vi "Get Ordered Channels_Status_IO.vi"(8 "error in (no error)":errorcluster, 11 "IO in":refnum<class "IO.lvclass">) -> (0 "error out":errorcluster, 1 "Ordered ICP2-DI Channels":T3[](array[typedef]), 2 "Ordered ICP2-DO Channels":T2[](array[typedef]), 3 "IO out":refnum<class "IO.lvclass">, 4 "Ordered ICP1-DO Channels":T1[](array[typedef]))   [LabVIEW 2022 SP3]
uses:
  IO.lvclass
  Typedefs/ICP2-DO Channel Names.ctl
  Typedefs/ICP2-DI Channel Names.ctl
  Typedefs/ICP1-D0 Channel Names.ctl
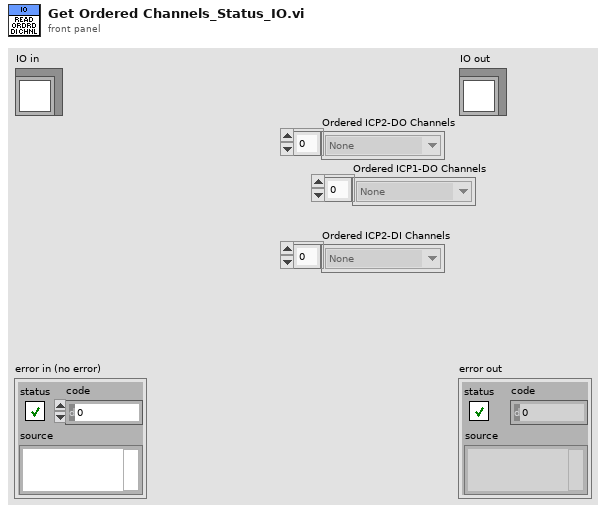
[diagram p1: front panel]
types:
  T1 = typedef "IO.lvclass/ICP1-D0 Channel Names.ctl" = enum16{"None", "Meniscus Pressure Reg PWR - R1", "Meniscus Pressure Reg PWR - R2", "Meniscus Pressure Reg PWR - R3", "Meniscus Pressure Reg PWR - R4", "Meniscus Pressure Reg PWR - R5", "Meniscus Pressure Reg PWR - R6", "Purge Valve Open - R1", "Purge Valve Open - R2", "Purge Valve Open - R3", "Purge Valve Open - R4", "Purge Valve Open - R5", "Purge Valve Open - R6"}
  T2 = typedef "IO.lvclass/ICP2-DO Channel Names.ctl" = enum16{"None", "Meniscus Valve Open - R1", "Meniscus Valve Open - R2", "Meniscus Valve Open - R3", "Meniscus Valve Open - R4", "Meniscus Valve Open - R5", "Meniscus Valve Open - R6", "Ink Flow Valve Open - R1", "Ink Flow Valve Open - R2", "Ink Flow Valve Open - R3", "Ink Flow Valve Open - R4", "Ink Flow Valve Open - R5", "Ink Flow Valve Open - R6", "SW_LED - Ink Valve - R1", "SW_LED - Ink Valve - R2", "SW_LED - Ink Valve - R3", "Recirc Pump On - R1", "Recirc Pump On - R2", "Recirc Pump On - R3", "Recirc Pump On - R4", "Recirc Pump On - R5", "Recirc Pump On - R6", "SW_LED - Ink Valve - R4", "SW_LED - Ink Valve - R5", "SW_LED - Ink Valve - R6"}
  T3 = typedef "IO.lvclass/ICP2-DI Channel Names.ctl" = enum16{"None", "SW - Ink Valve - R1", "SW - Ink Valve - R2", "SW - Ink Valve - R3", "SW - Ink Valve - R4", "SW - Ink Valve - R5", "SW - Ink Valve - R6", "SW - COVER INPUT SIDE", "SW - COVER OUTPUT SIDE", "SW - Purge - R1", "SW - Purge - R2", "SW - Purge - R3", "SW - Purge - R4", "SW - Purge - R5", "SW - Purge - R6"}
  T4 = typedef "IO.lvclass/Private Data.ctl" = cluster{"UserEvents":T5, "All Dependencies":cluster{"Class References":refnum<class>[], "Class Names":string[]}, "Status":T6}
  T5 = typedef "IO.lvclass/UserEvents.ctl" = cluster{"API Incoming Event":refnum<user-event>, "API Executed Event":refnum<user-event>, "API Return Event":refnum<user-event>, "Status Changed Event":refnum<user-event>}
  T6 = typedef "IO.lvclass/Status Cluster.ctl" = cluster{"Device Data":variant, "Ordered ICP1-DO Channels":T1[], "Ordered ICP2-DI Channels":T3[], "Ordered ICP2-DO Channels":T2[], "Ordered ICP1-AI Channels":T7[], "Ordered ICP1-AO Channels":T8[], "Ordered ICP2-AO Channels":T9[]}
  T7 = typedef "IO.lvclass/ICP1-AI Channel Names.ctl" = enum16{"None", "Meniscus Pressure Read - R1", "Meniscus Pressure Read - R2", "Meniscus Pressure Read - R3", "Meniscus Pressure Read - R4", "Meniscus Pressure Read - R5", "Meniscus Pressure Read - R6", "Meniscus Pressure Set - R1", "Meniscus Pressure Set - R2", "Meniscus Pressure Set - R3", "Meniscus Pressure Set - R4", "Meniscus Pressure Set - R5", "Meniscus Pressure Set - R6"}
  T8 = typedef "IO.lvclass/ICP1-AO Channel Names.ctl" = enum16{"None", "Meniscus Pressure Set - R1", "Meniscus Pressure Set - R2", "Meniscus Pressure Set - R3", "Meniscus Pressure Set - R4", "Meniscus Pressure Set - R5", "Meniscus Pressure Set - R6"}
  T9 = typedef "IO.lvclass/ICP2-AO Channel Names.ctl" = enum16{"None", "Recirc Pump Flow Set - R1", "Recirc Pump Flow Set - R2", "Recirc Pump Flow Set - R3", "Recirc Pump Flow Set - R4", "Recirc Pump Flow Set - R5", "Recirc Pump Flow Set - R6"}
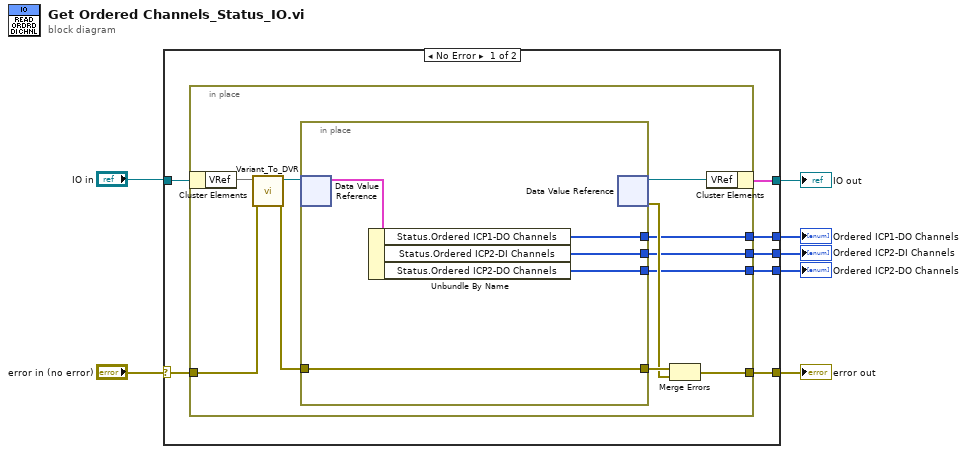
[diagram p0: block diagram]
diagram:
  n1 = case shown="No Error" "error in (no error)" {
    selector: "error in (no error)" -> [w11 w32]
    tunnel: [w13 w32] -> w5
    tunnel: [w14 w31] -> w4
    tunnel: "IO in" -> [w12 w31]
    tunnel: [w10 _] -> w3
    tunnel: [w9 _] -> w2
    tunnel: [w8 _] -> w1
    frame No Error {
      n2 = in-place {
        in-place-border: w11 -> [w23]
        in-place-border: [w19] -> w13
        in-place-border: [w17] -> w10
        in-place-border: [w16] -> w9
        in-place-border: [w15] -> w8
        n3 = in-place-cluster #1(w12) -> ("VRef"=w25)
        n4 = call "Variant_To_DVR.vi"("error in (no error)"=w23, "Variant"=w25) -> ("error out"=w22:errorcluster, "DVR"=w24:refnum<data-value>)  [unwired: 8 in]
        n5 = in-place {
          in-place-border: w22 -> [w29]
          in-place-border: [w29] -> w21
          in-place-border: [w28] -> w17
          in-place-border: [w27] -> w16
          in-place-border: [w26] -> w15
          n6 = in-place-dvr #2(w24) -> (w30:T4)  [unwired: 1 out]
          n7 = Unbundle By Name(w30) -> ("Status.Ordered ICP1-DO Channels"=w26:T1[], "Status.Ordered ICP2-DI Channels"=w28:T3[], "Status.Ordered ICP2-DO Channels"=w27:T2[])
          n8 = in-place-dvr #2() -> (w18:refnum<data-value>, w20:errorcluster)  [unwired: 1 in]
        }
        n9 = Merge Errors(w21, w20) -> (w19:errorcluster)
        n10 = in-place-cluster #1("VRef"=w18) -> (w14:cluster{})
      }
    }
    frame Error {
    }
  }
  "error out" <- w5
  "IO out" <- w4
  "Ordered ICP2-DI Channels" <- w3
  "Ordered ICP2-DO Channels" <- w2
  "Ordered ICP1-DO Channels" <- w1
